vi "DriveReadEncoder.vi"(8 "error in":errorcluster, 11 "ModualNamePrefix":i32) -> (0 "error out":errorcluster, 2 "SWERVE_DRIVE_MODULE_POSITION":T1={"Distance"=0.0, "Angle"={"VALUE"=0.0, "COS"=1.0, "SIN"=0.0}, "P"=FALSE} {"Angle"."SIN" format="%13.4f"; "Angle"."COS" format="%13.4f"; "Angle"."VALUE" format="%13.4f"}, 3 "SWERVE_DRIVE_MODULE_STATE":T3={"Speed"=0.0, "Angle"={"VALUE"=0.0, "COS"=1.0, "SIN"=0.0}} {"Angle"."SIN" format="%13.4f"; "Angle"."COS" format="%13.4f"; "Angle"."VALUE" format="%13.4f"})   [LabVIEW 2023]
uses:
  <vilib>/Rock Robotics/Network Tables/NT Write Number.vi
  <vilib>/Rock Robotics/WPI/ThirdParty/JAS_Junk/TrajLib/Trajectory_Library.lvlib
  DriveGlobal.vi
  <vilib>/Rock Robotics/WPI/ThirdParty/Phoenix-LabVIEW/CANCoder/Get/CTRE_Phoenix_CANcoder_GetSensorData.vi
  <vilib>/Rock Robotics/WPI/ThirdParty/JAS_Junk/TrajLib/TypeDef/ROTATION2D.ctl
  <vilib>/Rock Robotics/WPI/ThirdParty/JAS_Junk/TrajLib/TypeDef/SWERVE_DRIVE_MODULE_STATE.ctl
  <vilib>/Rock Robotics/WPI/ThirdParty/JAS_Junk/TrajLib/TypeDef/SWERVE_DRIVE_MODULE_POSITION.ctl
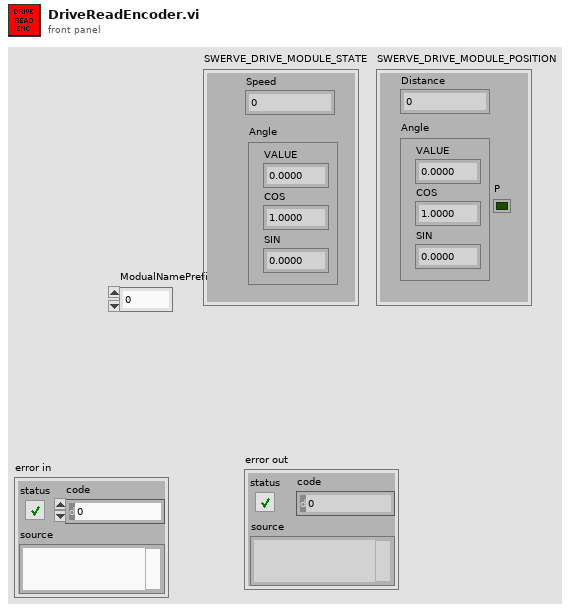
[diagram p1: front panel]
types:
  T1 = typedef "Trajectory_Library.lvlib/SWERVE_DRIVE_MODULE_POSITION.ctl" = cluster{"Distance":dbl, "Angle":T2, "P":bool}
  T2 = typedef "Trajectory_Library.lvlib/ROTATION2D.ctl" = cluster{"VALUE":dbl, "COS":dbl, "SIN":dbl}
  T3 = typedef "Trajectory_Library.lvlib/SWERVE_DRIVE_MODULE_STATE.ctl" = cluster{"Speed":dbl, "Angle":T2}
  T4 = typedef "WPI_MotorControlDeviceRef.ctl" = cluster{"DeviceStatus":errorcluster, "Type":T5, "PWM":cluster{"PWM Channel":T6, "DeadBand":T7}, "CAN":cluster{"Device Number":u8, "SetOutput VI Ref":variant, "GetOutput VI Ref":variant, "Enable VI Ref":variant, "Disable VI Ref":variant, "Data":variant}, "Invert":bool, "DIO PWM":cluster{"PWM \"Enable\" Channel":T6, "DIOChannel":T8, "PWM Rate":dbl}}
  T5 = typedef "WPI_MotorControlType.ctl" = enum16{"PWM", "CAN", "DIO PWM"}
  T6 = typedef "FPGA_DIOPWMChannel.ctl" = enum8{"PWM 0", "PWM 1", "PWM 2", "PWM 3", "PWM 4", "PWM 5", "PWM 6", "PWM 7", "PWM 8", "PWM 9", "PWM MXP 0", "PWM MXP 1", "PWM MXP 2", "PWM MXP 3", "PWM MXP 4", "PWM MXP 5", "PWM MXP 6", "PWM MXP 7", "PWM MXP 8", "PWM MXP 9", "Invalid"}
  T7 = typedef "WPI_PWMDeadband.ctl" = cluster{"Name":string, "maxPositivePwm":i32, "minPositivePwm":i32, "centerPwm":i32, "maxNegativePwm":i32, "minNegativePwm":i32, "angularRange":u16}
  T8 = typedef "FPGA_DIOChannel.ctl" = enum8{"DIO 0", "DIO 1", "DIO 2", "DIO 3", "DIO 4", "DIO 5", "DIO 6", "DIO 7", "DIO 8", "DIO 9", "DIO MXP 0", "DIO MXP 1", "DIO MXP 2", "DIO MXP 3", "DIO MXP 4", "DIO MXP 5", "DIO MXP 6", "DIO MXP 7", "DIO MXP 8", "DIO MXP 9", "DIO MXP 10", "DIO MXP 11", "DIO MXP 12", "DIO MXP 13", "DIO MXP 14", "DIO MXP 15", "SPI Port CS1", "SPI Port CS2", "SPI Port CS3", "SPI Port MISO", "SPI Port MOSI", "Invalid"}
  T9 = typedef "CTRE_Phoenix_CANcoder_DeviceRef.ctl" = cluster{"DeviceStatus":errorcluster, "Device Number":u8, "Handle":u64, "UsageFrame":u32, "Library Path":path}
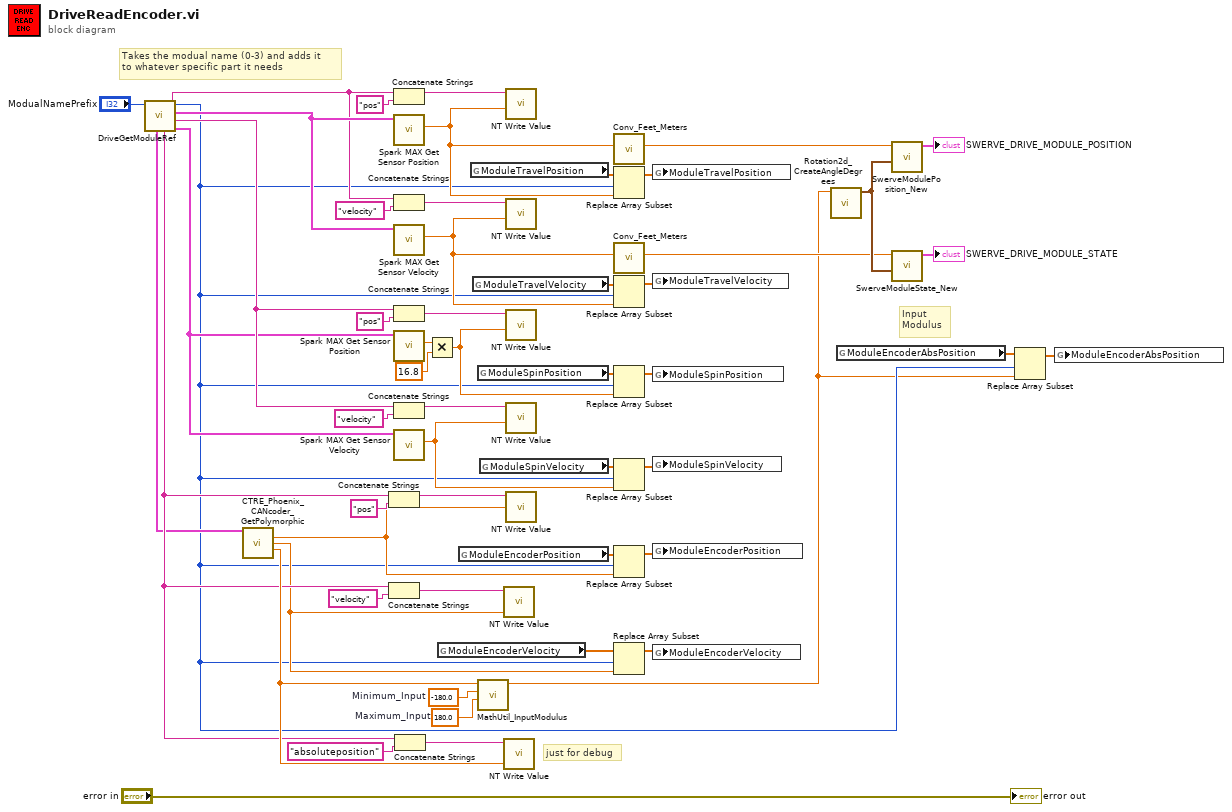
[diagram p0: block diagram]
diagram:
  w32 = -180.0  # Minimum_Input
  w31 = 180.0  # Maximum_Input
  # "Input\nModulus"
  # "just for debug"
  # "Takes the modual name (0-3) and adds it \nto whatever specific part it needs"
  n1 = call "DriveGetModuleRef.vi"("ModualNamePrefix"="ModualNamePrefix") -> ("SpinMot"=w22:T4, "SpinStr"=w24:string, "TravMot"=w42:T4, "TravStr"=w23:string, "EncStr"=w21:string, "EncDevice"=w20:T9)  [unwired: 5 in]
  n2 = call-poly <vilib>:"CTRE_Phoenix_CANcoder_GetPolymorphic.vi"("CTRE_CANcoder_DeviceRef"=w20) -> ("Position"=w8:dbl, "Velocity"=w5:dbl, "Absolute Position"=w30:dbl)  [unwired: 10 in, 2 out]
  n3 = Concatenate Strings(w21, "pos" ("refnum name")) -> (w51:string)
  n4 = Concatenate Strings(w21, "velocity" ("refnum name")) -> (w49:string)
  n5 = Concatenate Strings(w23, "pos" ("refnum name")) -> (w45:string)
  n6 = call <vilib>:"Spark MAX Get Sensor Position.vi"("MotorControlDevRef in"=w42) -> ("Sensor Position"=w25:dbl)  [unwired: 7 in, 3 out]
  n7 = Concatenate Strings(w23, "velocity" ("refnum name")) -> (w43:string)
  n8 = call <vilib>:"Spark MAX Get Sensor Velocity.vi"("MotorControlDevRef in"=w42) -> ("Sensor Velocity"=w17:dbl)  [unwired: 7 in, 3 out]
  n9 = Concatenate Strings(w24, "pos" ("refnum name")) -> (w40:string)
  n10 = call <vilib>:"Spark MAX Get Sensor Position.vi"("MotorControlDevRef in"=w22) -> ("Sensor Position"=w37:dbl)  [unwired: 7 in, 3 out]
  n11 = Concatenate Strings(w24, "velocity" ("refnum name")) -> (w38:string)
  n12 = call <vilib>:"Spark MAX Get Sensor Velocity.vi"("MotorControlDevRef in"=w22) -> ("Sensor Velocity"=w11:dbl)  [unwired: 7 in, 3 out]
  n13 = Concatenate Strings(w21, "absoluteposition" ("refnum name")) -> (w47:string)
  n14 = Multiply(x=w37, y=16.8) -> (x*y=w14:dbl)
  n15 = global read "DriveGlobal.vi" "ModuleEncoderVelocity"() -> (w7:dbl[])
  n16 = global read "DriveGlobal.vi" "ModuleEncoderPosition"() -> (w10:dbl[])
  n17 = global read "DriveGlobal.vi" "ModuleTravelPosition"() -> (w27:dbl[])
  n18 = global read "DriveGlobal.vi" "ModuleTravelVelocity"() -> (w19:dbl[])
  n19 = global read "DriveGlobal.vi" "ModuleSpinPosition"() -> (w16:dbl[])
  n20 = call <vilib>:"MathUtil_InputModulus.vi"("Maximum_Input"=w31, "Minimum_Input"=w32, "Input"=w30) -> ("modulus"=w1:dbl)  [unwired: 8 in]
  n21 = global read "DriveGlobal.vi" "ModuleSpinVelocity"() -> (w13:dbl[])
  n22 = call-poly <vilib>:"NT Write Value.vi"("value"=w5, "name"=w49) -> ()  [unwired: 9 in, 1 out]
  n23 = call-poly <vilib>:"NT Write Value.vi"("value"=w30, "name"=w47) -> ()  [unwired: 9 in, 1 out]
  n24 = call-poly <vilib>:"NT Write Value.vi"("value"=w25, "name"=w45) -> ()  [unwired: 9 in, 1 out]
  n25 = call-poly <vilib>:"NT Write Value.vi"("value"=w17, "name"=w43) -> ()  [unwired: 9 in, 1 out]
  n26 = call-poly <vilib>:"NT Write Value.vi"("value"=w14, "name"=w40) -> ()  [unwired: 9 in, 1 out]
  n27 = call-poly <vilib>:"NT Write Value.vi"("value"=w11, "name"=w38) -> ()  [unwired: 9 in, 1 out]
  n28 = call-poly <vilib>:"NT Write Value.vi"("value"=w8, "name"=w51) -> ()  [unwired: 9 in, 1 out]
  n29 = call <vilib>:"Conv_Feet_Meters.vi"("Feet"=w25) -> ("Meters"=w28:dbl)  [unwired: 10 in]
  n30 = Replace Array Subset(array=w27, new element=w25, index="ModualNamePrefix") -> (w26:dbl[])
  n31 = call <vilib>:"Conv_Feet_Meters.vi"("Feet"=w17) -> ("Meters"=w29:dbl)  [unwired: 10 in]
  n32 = Replace Array Subset(array=w19, new element=w17, index="ModualNamePrefix") -> (w18:dbl[])
  n33 = Replace Array Subset(array=w16, new element=w14, index="ModualNamePrefix") -> (w15:dbl[])
  n34 = Replace Array Subset(array=w13, new element=w11, index="ModualNamePrefix") -> (w12:dbl[])
  n35 = Replace Array Subset(array=w10, new element=w8, index="ModualNamePrefix") -> (w9:dbl[])
  n36 = Replace Array Subset(array=w7, new element=w5, index="ModualNamePrefix") -> (w6:dbl[])
  n37 = global write "DriveGlobal.vi" "ModuleTravelPosition"(w26) -> ()
  n38 = global write "DriveGlobal.vi" "ModuleTravelVelocity"(w18) -> ()
  n39 = global write "DriveGlobal.vi" "ModuleSpinPosition"(w15) -> ()
  n40 = global write "DriveGlobal.vi" "ModuleSpinVelocity"(w12) -> ()
  n41 = global write "DriveGlobal.vi" "ModuleEncoderPosition"(w9) -> ()
  n42 = global write "DriveGlobal.vi" "ModuleEncoderVelocity"(w6) -> ()
  n43 = call <vilib>:"Rotation2d_CreateAngleDegrees.vi"("Angle_Degrees"=w1) -> ("ROTATION"=w35:T2)  [unwired: 10 in]
  n44 = global read "DriveGlobal.vi" "ModuleEncoderAbsPosition"() -> (w4:dbl[])
  n45 = call <vilib>:"SwerveModulePosition_New.vi"("ROTATION"=w35, "Distance"=w28) -> ("SWERVE_DRIVE_MODULE_POSITION"=→"SWERVE_DRIVE_MODULE_POSITION":T1)  [unwired: 9 in]
  n46 = call <vilib>:"SwerveModuleState_New.vi"("ROTATION"=w35, "Speed"=w29) -> ("SWERVE_DRIVE_MODULE_STATE"=→"SWERVE_DRIVE_MODULE_STATE":T3)  [unwired: 9 in]
  n47 = Replace Array Subset(array=w4, new element=w1, index="ModualNamePrefix") -> (w3:dbl[])
  n48 = global write "DriveGlobal.vi" "ModuleEncoderAbsPosition"(w3) -> ()
  "error out" <- "error in"
